vi "Close & Abort VIs.vi"(8 "Error In":errorcluster, 11 "VI Paths":path[](array[path])) -> (0 "Error Out":errorcluster)   [LabVIEW 2019]
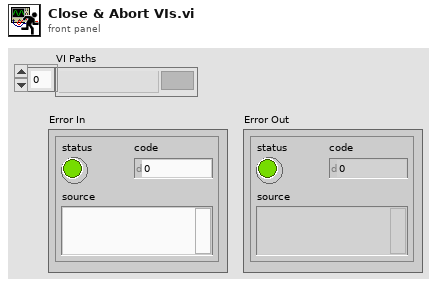
[diagram p1: front panel]
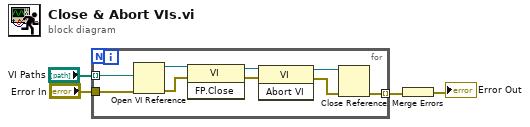
[diagram p0: block diagram]
diagram:
  n1 = for {
    tunnel: "VI Paths" -> [w13] mode=indexing
    tunnel: "Error In" -> [w6]
    tunnel: [w5] -> w2 mode=indexing
    n2 = Open VI Reference(vi path=w13, error in (no error)=w6) -> (vi reference=w12:refnum<vi>, error out=w11:errorcluster)  [unwired: 4 in]
    n3 = invoke class="VI" method="FP.Close"(reference=w12, error in=w11) -> (reference out=w10:refnum<vi>, error out=w9:errorcluster)  [unwired: 1 in, 1 out]
    n4 = invoke class="VI" method="Abort VI"(reference=w10, error in=w9) -> (reference out=w8:refnum<vi>, error out=w7:errorcluster)  [unwired: 1 in, 1 out]
    n5 = Close Reference(reference=w8, error in (no error)=w7) -> (error out=w5:errorcluster)
  }
  n6 = Merge Errors(w2) -> (→"Error Out":errorcluster)
